vi "Auton_S1_Right_Scale_2Cube.vi"   [LabVIEW 2017]
uses:
  <vilib>/Rock Robotics/WPI/Utilities/WPI_GetSetVariantRefNum.vi
  Robot Global Data.vi
  <vilib>/Rock Robotics/WPI/RobotDrive/WPI_RobotDriveArcadeDrive_Standard(NoSaturation).vi
types:
  T1 = typedef "WPI_RobotDriveDevRef.ctl" = cluster{"DevStatus":errorcluster, "Motors[]":T2[], "Square Inputs":bool, "Max Output":dbl}
  T2 = typedef "WPI_MotorControlDeviceRef.ctl" = cluster{"DeviceStatus":errorcluster, "Type":T3, "PWM":cluster{"PWM Channel":T4, "DeadBand":T5}, "CAN":cluster{"Device Number":u8, "SetOutput VI Ref":variant, "GetOutput VI Ref":variant, "Enable VI Ref":variant, "Disable VI Ref":variant, "Data":variant}, "Invert":bool, "DIO PWM":cluster{"PWM \"Enable\" Channel":T4, "DIOChannel":T6, "PWM Rate":dbl}}
  T3 = typedef "WPI_MotorControlType.ctl" = enum16{"PWM", "CAN", "DIO PWM"}
  T4 = typedef "FPGA_DIOPWMChannel.ctl" = enum8{"PWM 0", "PWM 1", "PWM 2", "PWM 3", "PWM 4", "PWM 5", "PWM 6", "PWM 7", "PWM 8", "PWM 9", "PWM MXP 0", "PWM MXP 1", "PWM MXP 2", "PWM MXP 3", "PWM MXP 4", "PWM MXP 5", "PWM MXP 6", "PWM MXP 7", "PWM MXP 8", "PWM MXP 9", "Invalid"}
  T5 = typedef "WPI_PWMDeadband.ctl" = cluster{"Name":string, "maxPositivePwm":i32, "minPositivePwm":i32, "centerPwm":i32, "maxNegativePwm":i32, "minNegativePwm":i32, "angularRange":u16}
  T6 = typedef "FPGA_DIOChannel.ctl" = enum8{"DIO 0", "DIO 1", "DIO 2", "DIO 3", "DIO 4", "DIO 5", "DIO 6", "DIO 7", "DIO 8", "DIO 9", "DIO MXP 0", "DIO MXP 1", "DIO MXP 2", "DIO MXP 3", "DIO MXP 4", "DIO MXP 5", "DIO MXP 6", "DIO MXP 7", "DIO MXP 8", "DIO MXP 9", "DIO MXP 10", "DIO MXP 11", "DIO MXP 12", "DIO MXP 13", "DIO MXP 14", "DIO MXP 15", "SPI Port CS1", "SPI Port CS2", "SPI Port CS3", "SPI Port MISO", "SPI Port MOSI", "Invalid"}
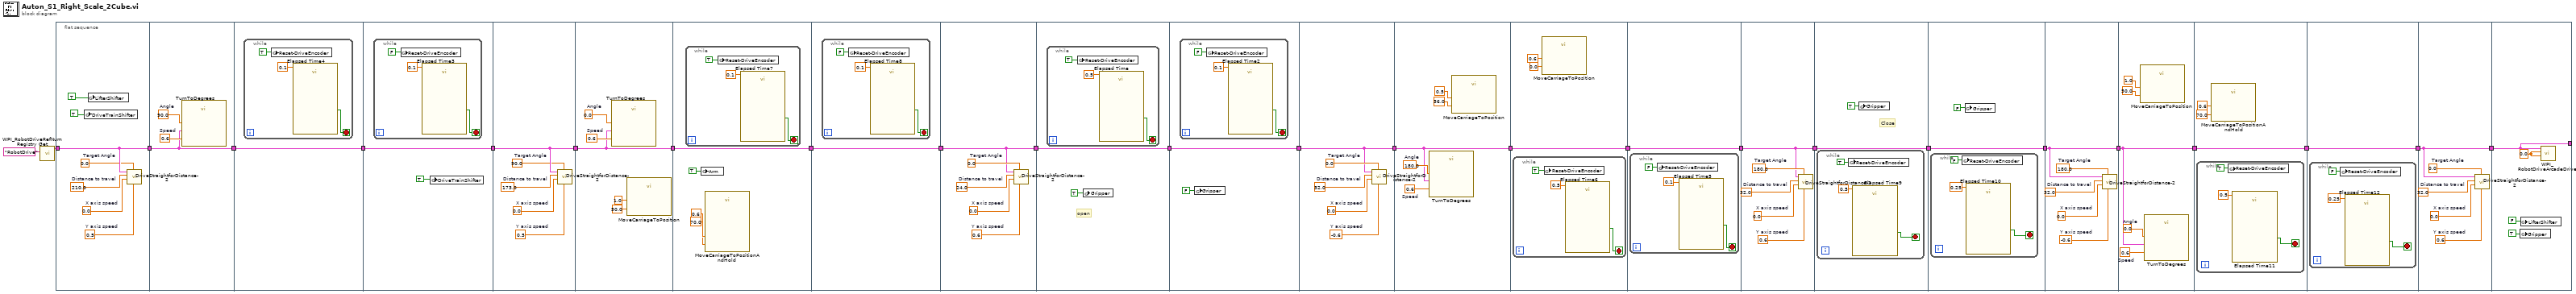
[diagram p0: block diagram]
diagram:
  n1 = call <vilib>:"WPI_RobotDriveRefNum Registry Get.vi"("refnum name"="RobotDrive") -> ("RobotDriveDevRef"=w24:T1)  [unwired: 9 in, 1 out]
  n2 = flat-sequence {
    tunnel: [w32] -> w21
    tunnel: w24 -> [w32]
    tunnel: w21 -> [w34]
    tunnel: [w34] -> w20
    tunnel: w20 -> [w36]
    tunnel: [w36] -> w22
    tunnel: w22 -> [w41]
    tunnel: [w41] -> w23
    tunnel: [w49] -> w19
    tunnel: w23 -> [w49]
    tunnel: w19 -> [w52]
    tunnel: [w52] -> w18
    tunnel: w18 -> [w58]
    tunnel: [w58] -> w17
    tunnel: w17 -> [w62]
    tunnel: [w62] -> w16
    tunnel: w16 -> [w66]
    tunnel: [w66] -> w15
    tunnel: w15 -> [w72]
    tunnel: [w72] -> w14
    tunnel: w14 -> [w77]
    tunnel: [w77] -> w13
    tunnel: w13 -> [w81]
    tunnel: [w81] -> w12
    tunnel: w12 -> [w88]
    tunnel: [w88] -> w11
    tunnel: w11 -> [w93]
    tunnel: [w93] -> w10
    tunnel: w10 -> [w97]
    tunnel: [w97] -> w9
    tunnel: w9 -> [w101]
    tunnel: [w101] -> w8
    tunnel: w8 -> [w107]
    tunnel: [w107] -> w7
    tunnel: w7 -> [w112]
    tunnel: [w112] -> w6
    tunnel: w6 -> [w116]
    tunnel: [w116] -> w5
    tunnel: w5 -> [w121]
    tunnel: [w121] -> w4
    tunnel: w4 -> [w128]
    tunnel: [w128] -> w3
    tunnel: w3 -> [w132]
    tunnel: [w132] -> w2
    tunnel: w2 -> [w136]
    tunnel: [w136] -> w1
    tunnel: [w143] -> _
    tunnel: w1 -> [w143]
    frame #0 {
      w28 = 0.0  # Target Angle
      w29 = 0.5  # Y axis speed
      w30 = 0.0  # X axis speed
      w31 = 210.0  # Distance to travel
      n3 = global write "Robot Global Data.vi" "DriveTrainShifter"(TRUE ("Gripper")) -> ()
      n4 = global write "Robot Global Data.vi" "LifterShifter"(TRUE ("Gripper")) -> ()
      n5 = call "DriveStraightforDistance-2.vi"("Y axis speed"=w29, "Target Angle"=w28, "X axis speed"=w30, "Distance to travel"=w31, "RobotDriveDevRef"=w32) -> ()  [unwired: 7 in]
    }
    frame #1 {
      w33 = 90.0  # Angle
      w35 = 0.6  # Speed
      n6 = call "TurnToDegrees.vi"("Speed"=w35, "RobotDriveDevRef"=w34, "Angle"=w33) -> ()  [unwired: 9 in]
    }
    frame #2 {
      n7 = while {
        stop <- w39 stop-if-true
        n8 = global write "Robot Global Data.vi" "Reset-DriveEncoder"(TRUE ("Reset-DriveEncoder")) -> ()
        n9 = call "Elapsed Time4"("Time Target (s)"=0.1) -> ("Time has Elapsed"=w39:bool)  [unwired: 11 in, 7 out]
      }
    }
    frame #3 {
      n10 = while {
        stop <- w44 stop-if-true
        n11 = global write "Robot Global Data.vi" "Reset-DriveEncoder"(FALSE ("Reset-DriveEncoder")) -> ()
        n12 = call "Elapsed Time3"("Time Target (s)"=0.1) -> ("Time has Elapsed"=w44:bool)  [unwired: 11 in, 7 out]
      }
      n13 = global write "Robot Global Data.vi" "DriveTrainShifter"(TRUE ("Gripper")) -> ()
    }
    frame #4 {
      w45 = 90.0  # Target Angle
      w46 = 0.5  # Y axis speed
      w47 = 0.0  # X axis speed
      w48 = 173.0  # Distance to travel
      n14 = call "DriveStraightforDistance-2.vi"("Y axis speed"=w46, "Target Angle"=w45, "X axis speed"=w47, "Distance to travel"=w48, "RobotDriveDevRef"=w49) -> ()  [unwired: 7 in]
    }
    frame #5 {
      w53 = 0.0  # Angle
      w54 = 0.6  # Speed
      n15 = call "TurnToDegrees.vi"("Speed"=w54, "RobotDriveDevRef"=w52, "Angle"=w53) -> ()  [unwired: 9 in]
      n16 = call "MoveCarriageToPosition.vi"("Lift Speed"=1.0, "Target Height"=50.0) -> ()  [unwired: 10 in]
    }
    frame #6 {
      n17 = while {
        stop <- w61 stop-if-true
        n18 = global write "Robot Global Data.vi" "Reset-DriveEncoder"(TRUE ("Reset-DriveEncoder")) -> ()
        n19 = call "Elapsed Time7"("Time Target (s)"=0.1) -> ("Time has Elapsed"=w61:bool)  [unwired: 11 in, 7 out]
      }
      n20 = global write "Robot Global Data.vi" "Arm"(TRUE ("Arm")) -> ()
      n21 = call "MoveCarriageToPositionAndHold.vi"("Lift Speed"=0.6, "Target Height"=70.0) -> ()  [unwired: 10 in]
    }
    frame #7 {
      n22 = while {
        stop <- w65 stop-if-true
        n23 = global write "Robot Global Data.vi" "Reset-DriveEncoder"(FALSE ("Reset-DriveEncoder")) -> ()
        n24 = call "Elapsed Time8"("Time Target (s)"=0.1) -> ("Time has Elapsed"=w65:bool)  [unwired: 11 in, 7 out]
      }
    }
    frame #8 {
      w67 = 0.0  # Target Angle
      w68 = 0.6  # Y axis speed
      w69 = 0.0  # X axis speed
      w70 = 24.0  # Distance to travel
      n25 = call "DriveStraightforDistance-2.vi"("Y axis speed"=w68, "Target Angle"=w67, "X axis speed"=w69, "Distance to travel"=w70, "RobotDriveDevRef"=w66) -> ()  [unwired: 7 in]
    }
    frame #9 {
      # "open"
      n26 = while {
        stop <- w75 stop-if-true
        n27 = global write "Robot Global Data.vi" "Reset-DriveEncoder"(TRUE ("Reset-DriveEncoder")) -> ()
        n28 = call "Elapsed Time"("Time Target (s)"=0.5) -> ("Time has Elapsed"=w75:bool)  [unwired: 11 in, 7 out]
      }
      n29 = global write "Robot Global Data.vi" "Gripper"(TRUE ("Gripper")) -> ()
    }
    frame #10 {
      n30 = while {
        stop <- w80 stop-if-true
        n31 = global write "Robot Global Data.vi" "Reset-DriveEncoder"(FALSE ("Reset-DriveEncoder")) -> ()
        n32 = call "Elapsed Time2"("Time Target (s)"=0.1) -> ("Time has Elapsed"=w80:bool)  [unwired: 11 in, 7 out]
      }
      n33 = global write "Robot Global Data.vi" "Gripper"(FALSE ("Gripper")) -> ()
    }
    frame #11 {
      w82 = 0.0  # Target Angle
      w83 = -0.6  # Y axis speed
      w84 = 0.0  # X axis speed
      w85 = 32.0  # Distance to travel
      n34 = call "DriveStraightforDistance-2.vi"("Y axis speed"=w83, "Target Angle"=w82, "X axis speed"=w84, "Distance to travel"=w85, "RobotDriveDevRef"=w81) -> ()  [unwired: 7 in]
    }
    frame #12 {
      w89 = 180.0  # Angle
      w90 = 0.6  # Speed
      n35 = call "TurnToDegrees.vi"("Speed"=w90, "RobotDriveDevRef"=w88, "Angle"=w89) -> ()  [unwired: 9 in]
      n36 = call "MoveCarriageToPosition.vi"("Lift Speed"=0.5, "Target Height"=36.0) -> ()  [unwired: 10 in]
    }
    frame #13 {
      n37 = while {
        stop <- w96 stop-if-true
        n38 = global write "Robot Global Data.vi" "Reset-DriveEncoder"(TRUE ("Reset-DriveEncoder")) -> ()
        n39 = call "Elapsed Time6"("Time Target (s)"=0.5) -> ("Time has Elapsed"=w96:bool)  [unwired: 11 in, 7 out]
      }
      n40 = call "MoveCarriageToPosition.vi"("Lift Speed"=0.6, "Target Height"=0.0) -> ()  [unwired: 10 in]
    }
    frame #14 {
      n41 = while {
        stop <- w100 stop-if-true
        n42 = global write "Robot Global Data.vi" "Reset-DriveEncoder"(FALSE ("Reset-DriveEncoder")) -> ()
        n43 = call "Elapsed Time5"("Time Target (s)"=0.1) -> ("Time has Elapsed"=w100:bool)  [unwired: 11 in, 7 out]
      }
    }
    frame #15 {
      w102 = 180.0  # Target Angle
      w103 = 0.6  # Y axis speed
      w104 = 0.0  # X axis speed
      w105 = 32.0  # Distance to travel
      n44 = call "DriveStraightforDistance-2.vi"("Y axis speed"=w103, "Target Angle"=w102, "X axis speed"=w104, "Distance to travel"=w105, "RobotDriveDevRef"=w101) -> ()  [unwired: 7 in]
    }
    frame #16 {
      # "Close"
      n45 = while {
        stop <- w110 stop-if-true
        n46 = global write "Robot Global Data.vi" "Reset-DriveEncoder"(TRUE ("Reset-DriveEncoder")) -> ()
        n47 = call "Elapsed Time9"("Time Target (s)"=0.5) -> ("Time has Elapsed"=w110:bool)  [unwired: 11 in, 7 out]
      }
      n48 = global write "Robot Global Data.vi" "Gripper"(TRUE ("Gripper")) -> ()
    }
    frame #17 {
      n49 = while {
        stop <- w115 stop-if-true
        n50 = global write "Robot Global Data.vi" "Reset-DriveEncoder"(FALSE ("Reset-DriveEncoder")) -> ()
        n51 = call "Elapsed Time10"("Time Target (s)"=0.25) -> ("Time has Elapsed"=w115:bool)  [unwired: 11 in, 7 out]
      }
      n52 = global write "Robot Global Data.vi" "Gripper"(FALSE ("Gripper")) -> ()
    }
    frame #18 {
      w117 = 180.0  # Target Angle
      w118 = -0.6  # Y axis speed
      w119 = 0.0  # X axis speed
      w120 = 32.0  # Distance to travel
      n53 = call "DriveStraightforDistance-2.vi"("Y axis speed"=w118, "Target Angle"=w117, "X axis speed"=w119, "Distance to travel"=w120, "RobotDriveDevRef"=w116) -> ()  [unwired: 7 in]
    }
    frame #19 {
      w122 = 0.0  # Angle
      w123 = 0.6  # Speed
      n54 = call "MoveCarriageToPosition.vi"("Lift Speed"=1.0, "Target Height"=50.0) -> ()  [unwired: 10 in]
      n55 = call "TurnToDegrees.vi"("Speed"=w123, "RobotDriveDevRef"=w121, "Angle"=w122) -> ()  [unwired: 9 in]
    }
    frame #20 {
      n56 = while {
        stop <- w131 stop-if-true
        n57 = global write "Robot Global Data.vi" "Reset-DriveEncoder"(TRUE ("Reset-DriveEncoder")) -> ()
        n58 = call "Elapsed Time11"("Time Target (s)"=0.5) -> ("Time has Elapsed"=w131:bool)  [unwired: 11 in, 7 out]
      }
      n59 = call "MoveCarriageToPositionAndHold.vi"("Lift Speed"=0.6, "Target Height"=70.0) -> ()  [unwired: 10 in]
    }
    frame #21 {
      n60 = while {
        stop <- w135 stop-if-true
        n61 = global write "Robot Global Data.vi" "Reset-DriveEncoder"(FALSE ("Reset-DriveEncoder")) -> ()
        n62 = call "Elapsed Time12"("Time Target (s)"=0.25) -> ("Time has Elapsed"=w135:bool)  [unwired: 11 in, 7 out]
      }
    }
    frame #22 {
      w137 = 0.0  # Target Angle
      w138 = 0.6  # Y axis speed
      w139 = 0.0  # X axis speed
      w140 = 32.0  # Distance to travel
      n63 = call "DriveStraightforDistance-2.vi"("Y axis speed"=w138, "Target Angle"=w137, "X axis speed"=w139, "Distance to travel"=w140, "RobotDriveDevRef"=w136) -> ()  [unwired: 7 in]
    }
    frame #23 {
      w144 = 0.0 ("X axis value")
      n64 = global write "Robot Global Data.vi" "Gripper"(TRUE ("Gripper")) -> ()
      n65 = global write "Robot Global Data.vi" "LifterShifter"(FALSE ("Gripper")) -> ()
      n66 = call-poly <vilib>:"WPI_RobotDriveArcadeDrive.vi"("Y axis value"=w144, "X axis value"=w144, "RobotDriveDevRef"=w143) -> ()  [unwired: 6 in, 3 out]
    }
  }
